vi "Start.vi"(6 "ms timeout (if waiting)":i32=-1, 8 "error in (no error)":errorcluster, 9 "Wait Until Shutdown? (F)":bool, 11 "JKI SMO in":refnum<class "JKI SMO.lvclass">) -> (0 "error out":errorcluster, 3 "JKI SMO out":refnum<class "JKI SMO.lvclass">)   [LabVIEW 2013, in "JKI SMO.lvclass"]
doc: "In the default mode (when <b>Wait Until Shutdown?</b> is False), this method will start (launch asynchronously) the registered processes.\n\nIf <b>Wait Until Shutdown?</b> is True, then this method is blocking (process launch is synchronous) until either the stop method is invoked or <b>ms timeout</b> is reached.\n\nNote 01: This method is overridable by descendant\nNote 02: When overridden, Call Parent Method is required\n\n---------------------------------------------------------------\nJKI State Machine Objects™\nhttp://jki.net/state-machine-objects/\nCopyright (C) 2005-2015, JKI <info@jki.net>\nALL RIGHTS RESERVED"
uses:
  JKI SMO.lvclass
  JKI SMO.lvclass/JKI SMO.ctl
  <vilib>/Utility/error.llb/Error Cluster From Error Code.vi
  <vilib>/ErrorRing/Error Ring.xnode
panel:
  # "For instructions on how to use the JKI State Machine Objects, examples and video tutorials, visit:\nhttp://jki.net/state-machine-objects/\n\nJKI State Machine Objects™\nhttp://jki.net/state-machine-objects/\nCopyright (C) 2005-2015, JKI <info@jki.net>\nALL RIGHTS RESERVED"
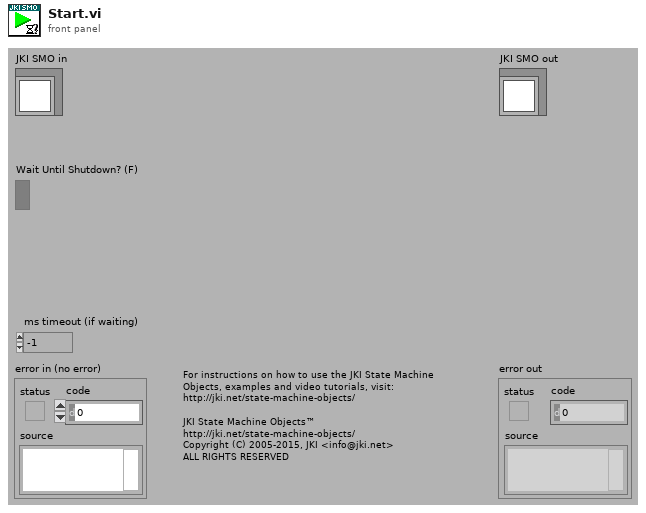
[diagram p1: front panel]
types:
  T1 = typedef "JKI SMO.lvclass/PrivateData--Cluster.ctl" = cluster{"Processes Clone VI Ref [ ]":refnum<vi>[], "Processes Clone Name [ ]":string[], "Process Sync RendezVous":T2, "Protected Events":T3, "Registered Process [ ]":T4[]}
  T2 = typedef "Rendezvous RefNum" = refnum<k1>
  T3 = typedef "JKI SMO.lvclass/ProtectedEvents--Cluster.ctl" = cluster{"StopProcesses":refnum<user-event>, "AbortProcesses":refnum<user-event>}
  T4 = typedef "JKI SMO.lvclass/RegisteredProcessData--Cluster.ctl" = cluster{"Name":string, "Static VI Ref":refnum<vi>}
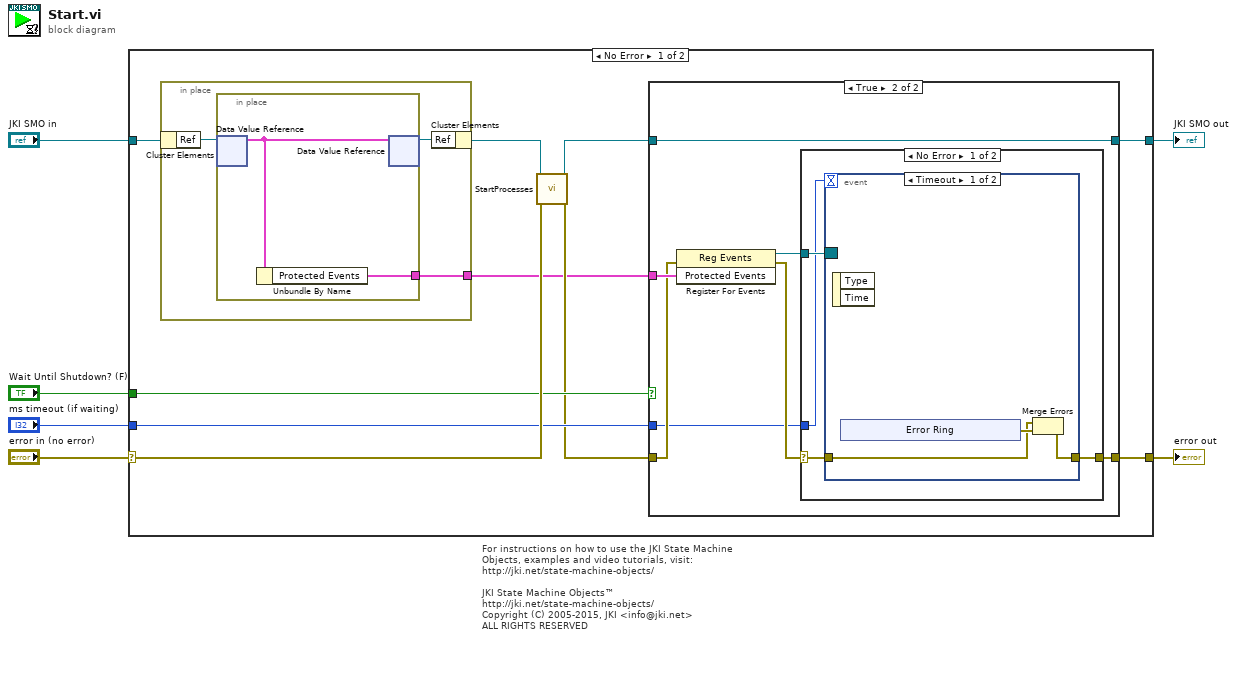
[diagram p0: block diagram]
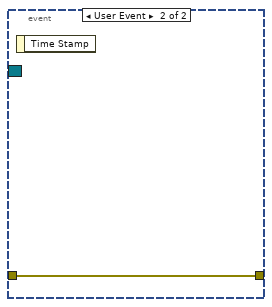
[diagram p3: hidden frame]
diagram:
  # "For instructions on how to use the JKI State Machine Objects, examples and video tutorials, visit:\nhttp://jki.net/state-machine-objects/\n\nJKI State Machine Objects™\nhttp://jki.net/state-machine-objects/\nCopyright (C) 2005-2015, JKI <info@jki.net>\nALL RIGHTS RESERVED"
  n1 = case shown="No Error" "error in (no error)" {
    selector: "error in (no error)" -> [w14 w45]
    tunnel: [w15 w45] -> w5
    tunnel: [w16 w44] -> w3
    tunnel: "JKI SMO in" -> [w13 w44]
    tunnel: "Wait Until Shutdown? (F)" -> [w12 _]
    tunnel: "ms timeout (if waiting)" -> [w11 _]
    frame No Error {
      n2 = in-place {
        in-place-border: [w39] -> w7
        n3 = in-place-cluster #1(w13) -> ("Ref"=w41:refnum<data-value>)
        n4 = in-place {
          in-place-border: [w43] -> w39
          n5 = in-place-dvr #2(w41) -> (w42:T1)  [unwired: 1 out]
          n6 = Unbundle By Name(w42) -> ("Protected Events"=w43:T3)
          n7 = in-place-dvr #2(w42) -> (w40:refnum<data-value>)  [unwired: 1 out]
        }
        n8 = in-place-cluster #1("Ref"=w40) -> (w10:refnum<class "JKI SMO.lvclass">)
      }
      n9 = call "StartProcesses.vi"("error in (no error)"=w14, "pSubSystem in"=w10) -> ("error out"=w8:errorcluster, "pSubSystem out"=w9:refnum<class "JKI SMO.lvclass">)  [unwired: 8 in]
      n10 = case shown="True" w12 {
        tunnel: w9 -> [w18 w21]
        tunnel: [w18 w21] -> w16
        tunnel: w8 -> [w17 w24]
        tunnel: [w17 w23] -> w15
        tunnel: w7 -> [_ w25]
        tunnel: w11 -> [_ w19]
        frame False {
        }
        frame True {
          n11 = register-events(error in=w24, w25) -> (reference out=w22:refnum<event-registration>, error out=w20:errorcluster)  [unwired: 1 in]
          n12 = case shown="No Error" w20 {
            selector: w20 -> [w27 w38]
            tunnel: [w29 w38] -> w23
            tunnel: w22 -> [w28 _]
            tunnel: w19 -> [w26 _]
            frame No Error {
              n13 = event shown="[0] Timeout" {
                selector: w28 -> [_ _]
                dyn-events: _ -> [_ _]
                timeout: w26 -> [_ _]
                tunnel: w27 -> [w31 w37]
                tunnel: [w30 w37] -> w29
                event Timeout {
                  n14 = event-data() -> ()  [unwired: 1 in, 2 out]
                  n15 = xnode "Error Ring"() -> ("error out"=w32:errorcluster)
                  n16 = Merge Errors(w31, w32) -> (w30:errorcluster)
                }
                event User Event {
                  n17 = event-data() -> ()  [unwired: 1 in, 1 out]
                }
              }
            }
            frame Error {
            }
          }
        }
      }
    }
    frame Error {
    }
  }
  "error out" <- w5
  "JKI SMO out" <- w3
